vi "time date.vi"() -> ()   [LabVIEW 2024]
panel:
  out "date/time string":string
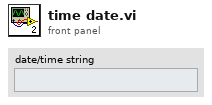
[diagram p1: front panel]
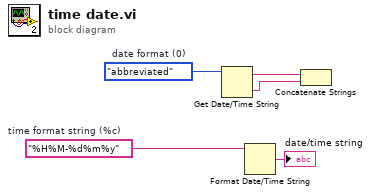
[diagram p0: block diagram]
diagram:
  w1 = "%H%M-%d%m%y"  # time format string (%c)
  w3 = enum16{"short", "long", "abbreviated"}."abbreviated"  # date format (0)
  n1 = Get Date/Time String(date format (0)=w3) -> (date string=w5:string, time string=w4:string)  [unwired: 2 in]
  n2 = Format Date/Time String(time format string (%c)=w1) -> (date/time string=→"date/time string":string)  [unwired: 2 in]
  n3 = Concatenate Strings(w5, w4) -> ()  [unwired: 1 out]
